vi "daqio_Get_All_Devices.vi"(8 "error in":errorcluster, 11 "daq.io type in":T4={"daq.io ref"=refnum, "daq.io API Base"="http://dashboard.daq.io/api/v1", "Device Key"="", "Account ID"="", "online"=TRUE, "SSL"=TRUE}) -> (0 "error out":errorcluster, 2 "Devices":T1[](array[typedef]), 3 "daq.io type out":T4={"daq.io ref"=refnum, "daq.io API Base"="http://dashboard.daq.io/api/v1", "Device Key"="", "Account ID"="", "online"=TRUE, "SSL"=TRUE})   [LabVIEW 2013, in "daqio minimal.lvlib"]
doc: "This VI returns all Devices associated with the logged in user on this account.\nThis returns a potentially large JSON document over the network. When only limited bandwidth is available, try more specific fucntions such as \"Get Specific Device Type\" or similar."
uses:
  daqio minimal.lvlib
  _typedefs/daqio-Type.ctl
  <vilib>/httpClient/ClientHandle.ctl
  _typedefs/daqio-Device.ctl
  _typedefs/daqio-Channels.ctl
  _typedefs/daqio-Device-Dashboards.ctl
  <vilib>/Easy HTTP Client/Easy HTTP.lvlib
  <vilib>/httpClient/LabVIEWHTTPClient.lvlib
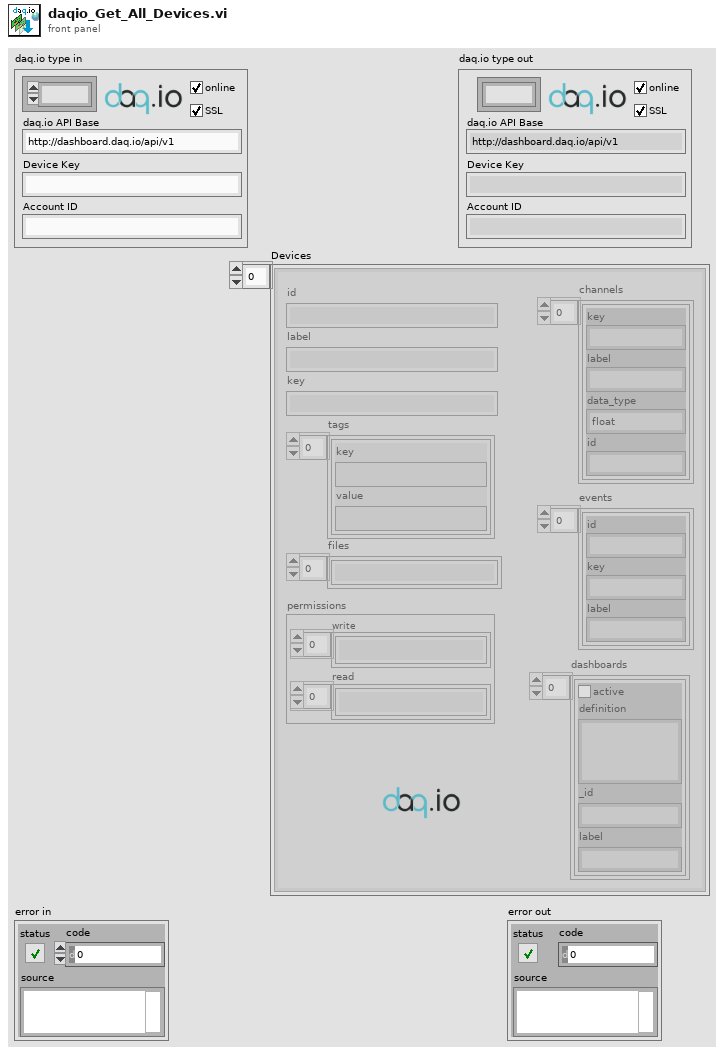
[diagram p1: front panel]
types:
  T1 = typedef "daqio minimal.lvlib/daqio-Device.ctl" = cluster{"id":string, "label":string, "key":string, "channels":T2[], "tags":cluster{"key":string, "value":string}[], "events":cluster{"id":string, "key":string, "label":string}[], "files":string[], "permissions":cluster{"write":string[], "read":string[]}, "dashboards":T3[]}
  T2 = typedef "daqio minimal.lvlib/daqio-Channels.ctl" = cluster{"key":string, "label":string, "data_type":string, "id":string}
  T3 = typedef "daqio minimal.lvlib/daqio-Device-Dashboards.ctl" = cluster{"active":bool, "definition":string, "_id":string, "label":string}
  T4 = typedef "daqio minimal.lvlib/daqio-Type.ctl" = cluster{"daq.io ref":T5, "daq.io API Base":string, "Device Key":string, "Account ID":string, "online":bool, "SSL":bool}
  T5 = typedef "LabVIEWHTTPClient.lvlib/ClientHandle.ctl" = refnum<k1>
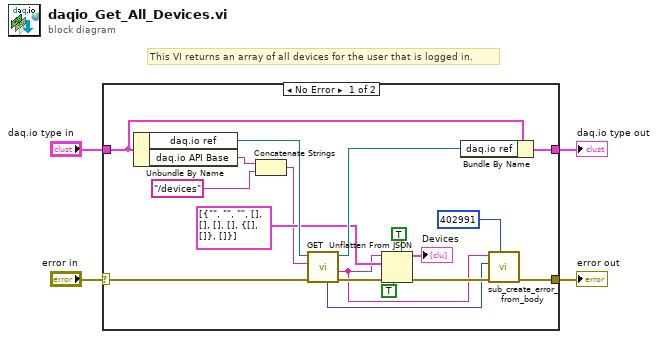
[diagram p0: block diagram]
diagram:
  # "This VI returns an array of all devices for the user that is logged in."
  n1 = case shown="No Error" "error in" {
    selector: "error in" -> [w18 w23]
    tunnel: "daq.io type in" -> [w22 w24]
    tunnel: [w21 w24] -> w3
    tunnel: [w9 w23] -> w2
    frame No Error {
      n2 = Unbundle By Name(w22) -> ("daq.io ref"=w20:T5, "daq.io API Base"=w16:string)
      n3 = Concatenate Strings(w16, "/devices") -> (w13:string)
      n4 = call <vilib>:"GET.vi"("error in (no error)"=w18, "url"=w13, "client handle"=w20) -> ("error out"=w17:errorcluster, "body"=w6:string, "client handle out"=w19:T5, "HTTP Response Code"=w8:i32)  [unwired: 4 in, 1 out]
      n5 = Unflatten From JSON(enable LabVIEW extensions? (T)=TRUE, JSON string=w6, type and defaults=T1[] [{"id"="", "label"="", "key"="", "channels"=[], "tags"=[], "events"=[], "files"=[], "permissions"={"write"=[], "read"=[]}, "dashboards"=[]}], default null elements? (F)=TRUE, error in (no error)=w17) -> (value=→"Devices":T1[], error out=w10:errorcluster)  [unwired: 2 in]
      n6 = Bundle By Name(cluster=w22, "daq.io ref"=w19) -> (w21:T4)
      n7 = call "sub_create_error_from_body.vi"("error code"=402991, "error in (no error)"=w10, "http code"=w8, "body"=w6) -> ("error out"=w9:errorcluster)  [unwired: 7 in]
    }
    frame Error {
    }
  }
  "error out" <- w2
  "daq.io type out" <- w3
